vi "S2C_ExeSearchStepGlobal.vi"(8 "Error In":errorcluster, 9 "Reset?":bool, 10 "ResultName":string, 11 "Command":string) -> (0 "Error Out":errorcluster, 2 "Found?":bool, 3 "Result Value":variant)   [LabVIEW 2015]
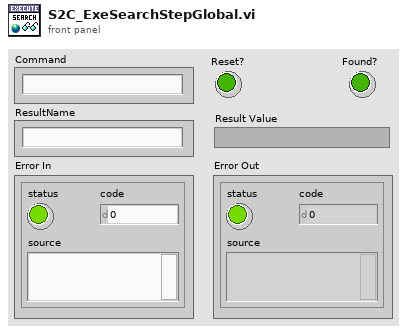
[diagram p1: front panel]
types:
  T1 = cluster{"Command":string, "Result Name":string, "Result Value":variant}[]
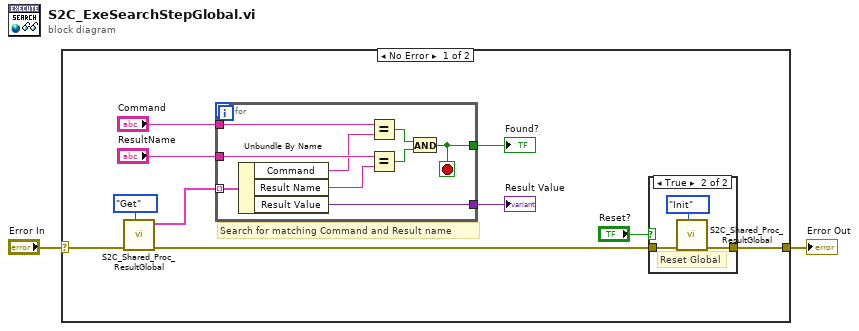
[diagram p0: block diagram]
diagram:
  n1 = case shown="No Error" "Error In" {
    selector: "Error In" -> [w12 w26]
    tunnel: [w5 w26] -> w1
    frame No Error {
      # "Search for matching Command and Result name"
      n2 = call "S2C_Shared_Proc_ResultGlobal.vi"("Action"=enum16{"Init", "Add", "Get"}."Get", "Error In"=w12) -> ("Error Out"=w6:errorcluster, "Data Out"=w10:T1)  [unwired: 8 in]
      n3 = for {
        tunnel: w10 -> [w20] mode=indexing
        tunnel: "ResultName" -> [w25]
        tunnel: "Command" -> [w24]
        tunnel: [w21] -> w7
        tunnel: [w17] -> w3
        stop <- w21 stop-if-true
        n4 = Unbundle By Name(w20) -> ("Command"=w19:string, "Result Name"=w18:string, "Result Value"=w17:variant)
        n5 = Equal?(x=w24, y=w19) -> (x = y?=w22:bool)
        n6 = Equal?(x=w25, y=w18) -> (x = y?=w23:bool)
        n7 = And(x=w22, y=w23) -> (x .and. y?=w21:bool)
      }
      "Found?" <- w7
      "Result Value" <- w3
      n8 = case shown="True" "Reset?" {
        tunnel: w6 -> [w13 w15]
        tunnel: [w13 w14] -> w5
        frame False {
        }
        frame True {
          # "Reset Global"
          n9 = call "S2C_Shared_Proc_ResultGlobal.vi"("Action"=enum16{"Init", "Add", "Get"}."Init", "Error In"=w15) -> ("Error Out"=w14:errorcluster)  [unwired: 8 in, 1 out]
        }
      }
    }
    frame Error {
    }
  }
  "Error Out" <- w1
